vi "min.vi"(9 "Numeric":dbl) -> (3 "Numeric 2":dbl format="%#_13g")   [LabVIEW 2022 SP3]
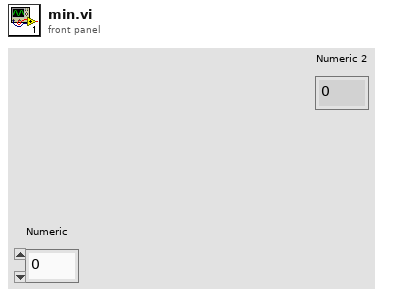
[diagram p1: front panel]
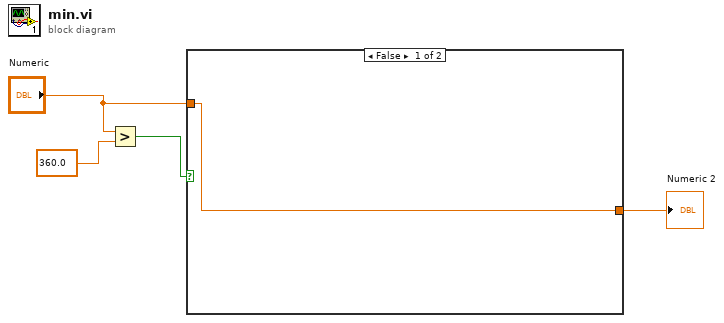
[diagram p0: block diagram]
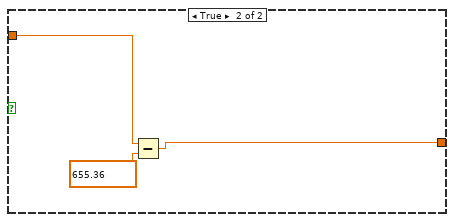
[diagram p2: hidden frame]
diagram:
  n1 = Greater?(x="Numeric", y=360.0) -> (0:w3:bool)
  n2 = case shown="False" w3 {
    tunnel: "Numeric" -> [w5 w7]
    tunnel: [w5 w6] -> w1
    frame False {
    }
    frame True {
      n3 = Subtract(x=w7, y=655.36) -> (x-y=w6:dbl)
    }
  }
  "Numeric 2" <- w1
